vi "DS1104PlusDemo.vi"() -> ()   [LabVIEW 2018]
uses:
  <vilib>/event_ctls.llb/usereventprio.ctl
panel:
  in  "GetCurrentStatus":bool
  in  "Exit":bool
  out "错误输出":errorcluster
  in  "接口类型":u16(ring)=1 items=[""=0, "GPIB"=1, "VXI"=2, "GPIB-VXI"=3, "Serial"=4, "PXI"=5, "TCPIP"=6, "USB"=7, "FireWire"=9]
  in  "SINGLE Trigger":bool
  in  "RUN/STOP":bool
  in  "AUTO Set":bool
  in  "CLEAR Display":bool
  in  "Vertical Coupling":u16(ring) items=["AC", "DC", "Ground"]
  in  "Probe Attenuation":u16(ring) items=["1x"=1, "10x"=10]
  out "Single":bool caption="SINGLE"
  out "Normal":bool caption="NORMAL"
  out "Auto":bool caption="AUTO"
  in  "Trigger MODE":string(combo)
  in  "FORCE Trigger":bool
  in  "Trigger MENU":bool
  in  "Trigger LEVEL":dbl step=0.01 format="%.6g"
  in  "Horizontal POSITION":ext format="%#_9g"
  in  "Horizontal MENU":bool
  in  "Horizaontal SCALE":ext(ring)=1e-09 items=["1u", "2u", "5u", "10u", "20u", "50u", "100u", "200u", "500u", "1m", "2m", "5m", "10m", "20m", "50m", "100m", "200m", "500m", "1", "2", "5", "10", "20", "50", "100", "200", "500", "1000"]
  in  "Vertical SCALE":dbl(ring) items=["500u"=0.0005, "1m"=0.001, "2m"=0.002, "5m"=0.005, "10m"=0.01, "20m"=0.02, "50m"=0.05, "100m"=0.1, "200m"=0.2, "500m"=0.5, "1"=1.0, "2"=2.0, "5"=5.0, "10"=10.0, "20"=20.0, "50"=50.0, "100"=100.0]
  in  "Vertical POSITION":dbl min=-100.0 max=100.0 step=0.1 format="%#_4g"
  in  "CH4":bool
  in  "CH3":bool
  in  "CH2":bool
  in  "CH1":bool
  out "波形图":waveform(dbl)[](graph)
  in  "VISA资源名称":refnum<visa-resource-name>
  # "VERTICAL"
  # "HORIZONTAL"
  # "TRIGGER"
  # "POSITION"
  # "POSITION"
  # "V"
  # "s"
  # "SCALE"
  # "SCALE"
  # "s/div"
  # "V/div"
  # "V"
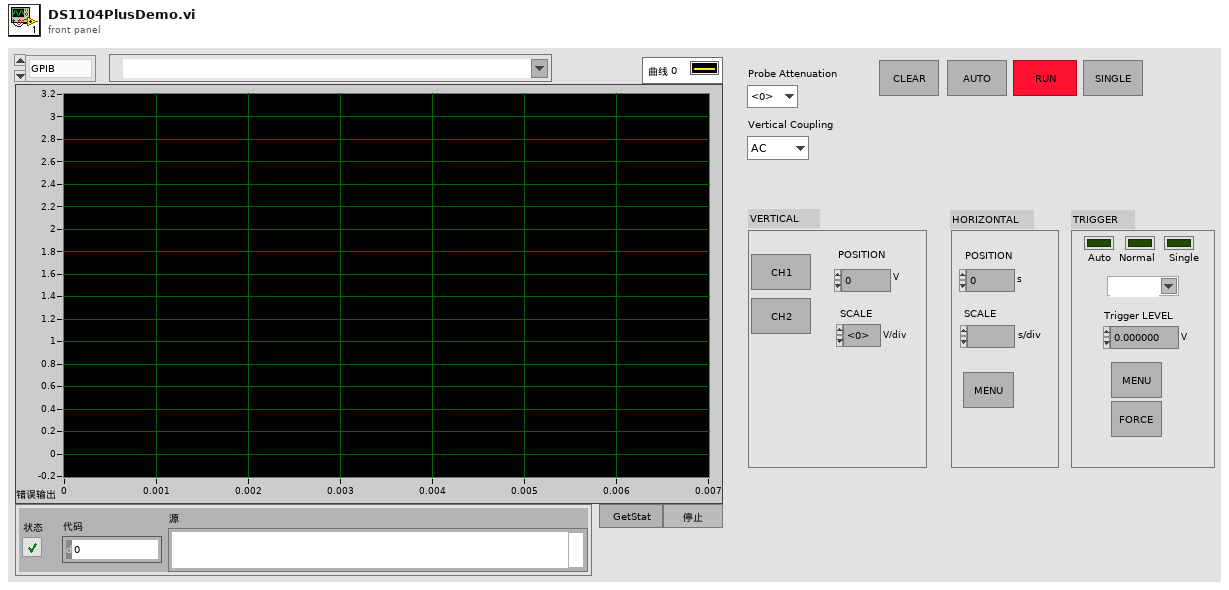
[diagram p1: front panel]
types:
  T1 = typedef "usereventprio.ctl" = enum32{"high priority", "normal priority"}
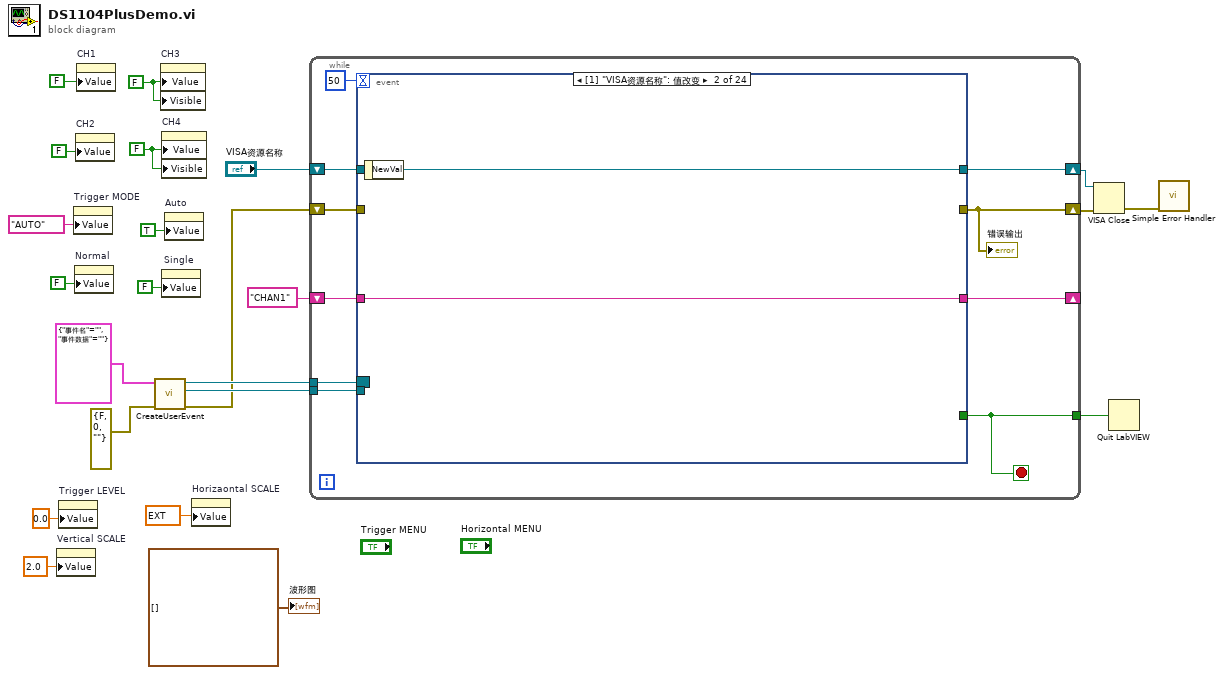
[diagram p0: block diagram]
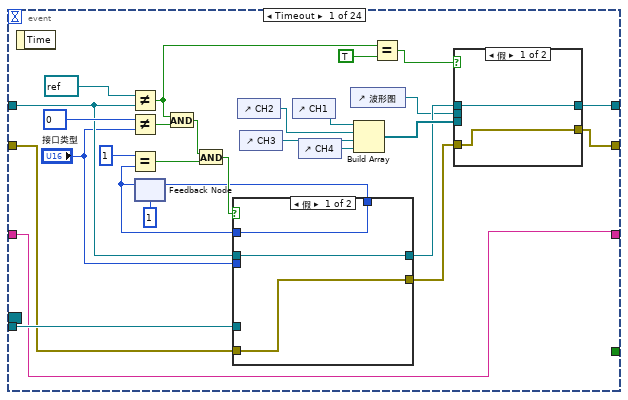
[diagram p2: hidden frame]
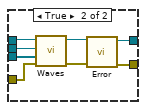
[diagram p3: hidden frame]
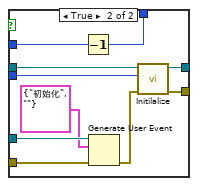
[diagram p4: hidden frame]
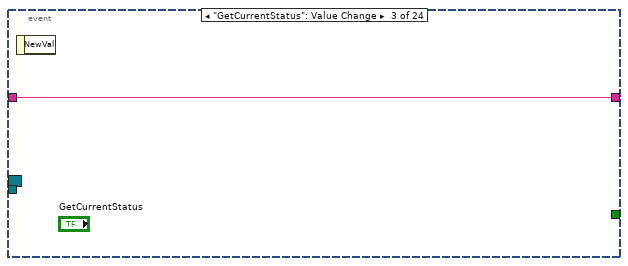
[diagram p5: hidden frame]
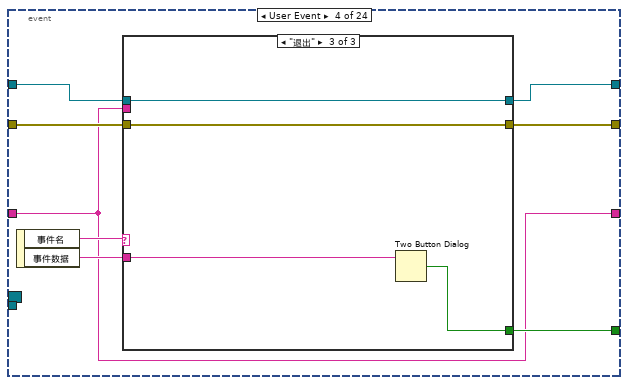
[diagram p6: hidden frame]
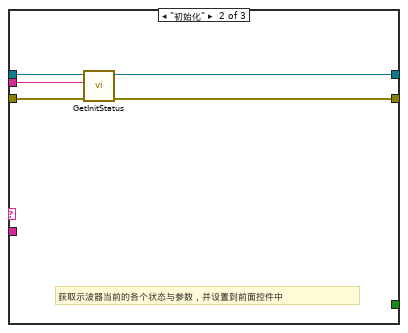
[diagram p8: hidden frame]
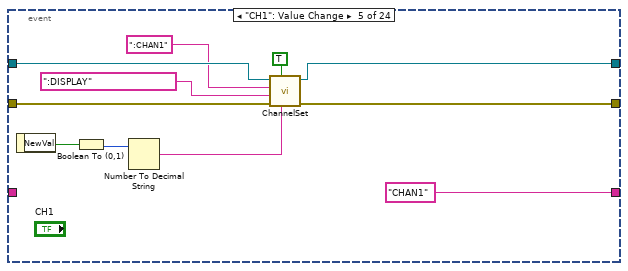
[diagram p9: hidden frame]
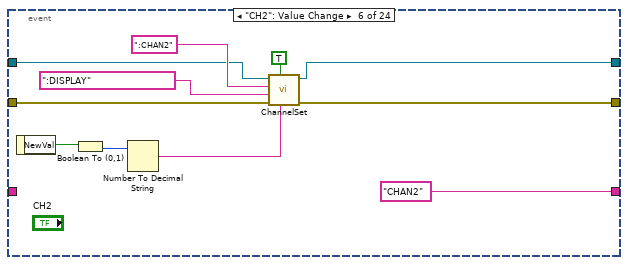
[diagram p10: hidden frame]
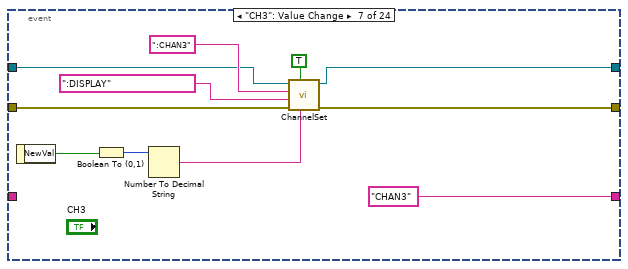
[diagram p11: hidden frame]
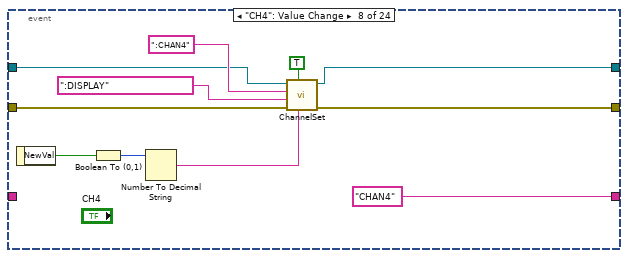
[diagram p12: hidden frame]
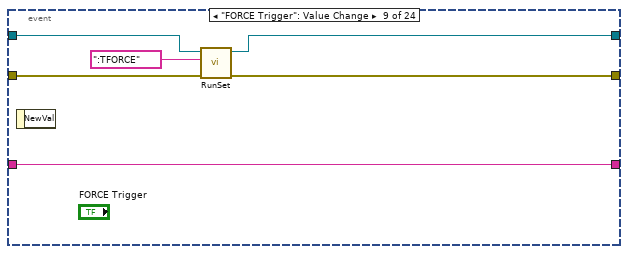
[diagram p13: hidden frame]
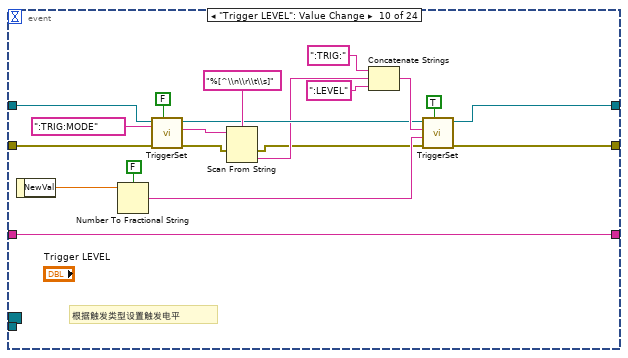
[diagram p14: hidden frame]
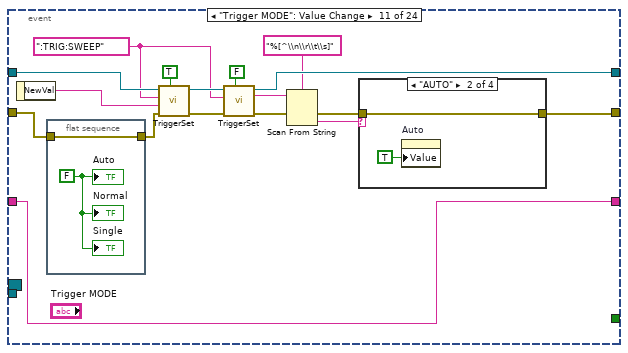
[diagram p15: hidden frame]
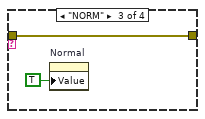
[diagram p17: hidden frame]
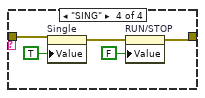
[diagram p18: hidden frame]
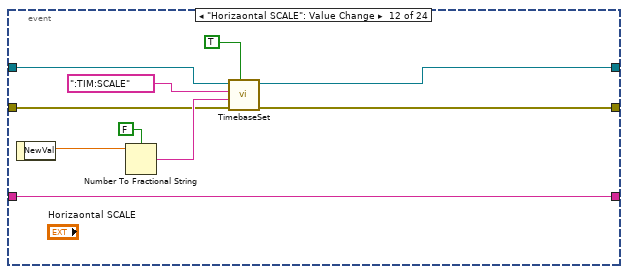
[diagram p19: hidden frame]
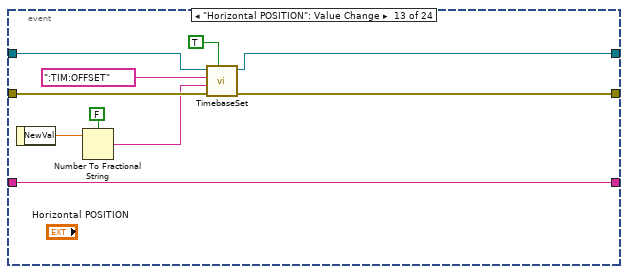
[diagram p20: hidden frame]
diagram:
  w5 = ext 0.00099999999999999999996 items=["1u", "2u", "5u", "10u", "20u", "50u", "100u", "200u", "500u", "1m", "2m", "5m", "10m", "20m", "50m", "100m", "200m", "500m", "1", "2", "5", "10", "20", "50", "100", "200", "500", "1000"] ("Horizaontal SCALE")
  w7 = 2.0 items=["500u"=0.0005, "1m"=0.001, "2m"=0.002, "5m"=0.005, "10m"=0.01, "20m"=0.02, "50m"=0.05, "100m"=0.1, "200m"=0.2, "500m"=0.5, "1"=1.0, "2"=2.0, "5"=5.0, "10"=10.0, "20"=20.0, "50"=50.0, "100"=100.0] ("Vertical SCALE")
  w8 = FALSE ("CH4")
  w9 = FALSE ("CH3")
  n1 = property on="Vertical SCALE" class="Ring (严格)"("Value"=w7) -> ()  [unwired: 2 in, 2 out]
  n2 = property on="Trigger LEVEL" class="DigNum (严格)"("Value"=0.0 ("Trigger LEVEL")) -> ()  [unwired: 2 in, 2 out]
  n3 = property on="Trigger MODE" class="CmbBox"("Value"="AUTO" ("Trigger MODE")) -> ()  [unwired: 2 in, 2 out]
  n4 = property on="Normal" class="Bool (严格)"("Value"=FALSE ("Normal")) -> ()  [unwired: 2 in, 2 out]
  n5 = property on="CH2" class="Bool (严格)"("Value"=FALSE ("CH2")) -> ()  [unwired: 2 in, 2 out]
  n6 = property on="CH1" class="Bool (严格)"("Value"=FALSE ("CH1")) -> ()  [unwired: 2 in, 2 out]
  n7 = call "CreateUserEvent.vi"("error in (no error)"=errorcluster {"status"=FALSE, "code"=0, "source"=""} ("错误常量"), "事件消息"=cluster{"事件名":string, "事件数据":string} {"事件名"="", "事件数据"=""}) -> ("error out"=w11:errorcluster, "用户事件引用句柄"=w13:refnum<user-event>, "用户事件注册引用句柄"=w14:refnum<event-registration>)  [unwired: 7 in]
  n8 = property on="CH3" class="Bool (严格)"("Value"=w9, "Visible"=w9) -> ()  [unwired: 2 in, 2 out]
  n9 = property on="CH4" class="Bool (严格)"("Value"=w8, "Visible"=w8) -> ()  [unwired: 2 in, 2 out]
  n10 = property on="Single" class="Bool (严格)"("Value"=FALSE ("Single")) -> ()  [unwired: 2 in, 2 out]
  n11 = property on="Auto" class="Bool (严格)"("Value"=TRUE ("Auto")) -> ()  [unwired: 2 in, 2 out]
  n12 = property on="Horizaontal SCALE" class="Ring (严格)"("Value"=w5) -> ()  [unwired: 2 in, 2 out]
  n13 = while {
    shift-right: [w27] -> w18
    shift-left: "VISA资源名称" -> [w32]
    shift-right: [w26] -> w17
    shift-left: w11 -> [w31]
    shift-right: [w29] -> _
    shift-left: "CHAN1" ("通道选择") -> [w30]
    tunnel: w14 -> [w25]
    tunnel: w13 -> [w28]
    tunnel: [w24] -> w1
    stop <- w24 stop-if-true
    n14 = event shown="[1] \"VISA资源名称\": 值改变" {
      selector: w25 -> [_ _ _ _ _ _ _ _ _ _ _ _ _ _ _ _ _ _ _ _ _ _ _ _]
      dyn-events: _ -> [_ _ _ _ _ _ _ _ _ _ _ _ _ _ _ _ _ _ _ _ _ _ _ _]
      timeout: 50 -> [_ _ _ _ _ _ _ _ _ _ _ _ _ _ _ _ _ _ _ _ _ _ _ _]
      tunnel: w32 -> [w46 _ _ w94 w117 w122 w135 w146 w154 w175 w193 w215 w224 w235 w243 w255 w261 w268 w274 w286 w320 w341 w358 w369]
      tunnel: w31 -> [w59 _ _ w90 w116 w121 w134 w145 w155 w174 w184 w209 w225 w226 w242 w253 w264 w267 w275 w285 w321 w340 w360 w368]
      tunnel: [w40 w85 _ w93 w109 w120 w133 w144 w151 w163 w185 w208 w219 w230 w238 w252 w262 w266 w273 w277 w315 w338 w358 w369] -> w27
      tunnel: [w37 _ _ w91 w108 w119 w132 w143 w153 w164 w186 w207 w218 w228 w237 w251 w263 w265 w272 w278 w317 w339 w359 w368] -> w26
      tunnel: w30 -> [w41 w86 w87 w88 _ _ _ _ w156 w176 w192 w206 w217 w231 w236 w249 w260 w270 w276 w287 w322 w343 w364 w370]
      tunnel: [w41 w86 w87 w88 "CHAN1" ("通道选择") "CHAN2" ("通道选择") "CHAN3" ("通道选择") "CHAN4" ("通道选择") w156 w176 w192 w206 w217 w231 w236 w249 w260 w270 w276 w287 w322 w342 w364 w370] -> w29
      tunnel: w28 -> [w60 _ _ _ _ _ _ _ _ _ _ _ _ _ _ _ _ _ _ _ _ w337 w361 _]
      tunnel: [_ _ _ w89 _ _ _ _ _ _ _ _ _ _ _ _ _ _ _ _ _ _ _ w365] -> w24
      event Timeout {
        w61 = u16 0 items=[""=0, "GPIB"=1, "VXI"=2, "GPIB-VXI"=3, "Serial"=4, "PXI"=5, "TCPIP"=6, "USB"=7, "FireWire"=9] ("接口类型")
        n15 = event-data() -> ()  [unwired: 1 in, 1 out]
        n16 = Not Equal?(x=refnum<visa-resource-name> refnum ("y"), y=w46) -> (x != y?=w35:bool)
        n17 = Not Equal?(x=w61, y="接口类型") -> (x != y?=w54:bool)
        n18 = feedback #1(1) -> (w56:i32)
        n19 = Equal?(x=1, y=w56) -> (x = y?=w53:bool)
        n20 = And(x=w35, y=w54) -> (x .and. y?=w44:bool)
        n21 = And(x=w44, y=w53) -> (x .and. y?=w52:bool)
        n22 = case shown="假" w52 {
          tunnel: w60 -> [_ w84]
          tunnel: w59 -> [w72 w82]
          tunnel: w56 -> [w74 w81]
          tunnel: [w74 w80] -> w47
          tunnel: w46 -> [w73 w79]
          tunnel: "接口类型" -> [_ w78]
          tunnel: [w73 w76] -> w42
          tunnel: [w72 w75] -> w38
          frame False {
          }
          frame True {
            n23 = Decrement(x=w81) -> (x-1=w80:i32)
            n24 = Generate User Event(user event=w84, event data cluster=cluster{"事件名":string, "事件数据":string} {"事件名"="初始化", "事件数据"=""} ("事件数据"), error in=w82) -> (error out=w77:errorcluster)  [unwired: 1 in, 1 out]
            n25 = call "Initilalize.vi"("错误输入（无错误）"=w77, "接口类型"=w78, "VISA资源名称"=w79) -> ("错误输出"=w75:errorcluster, "VISA资源名称输出"=w76:refnum<visa-resource-name>)  [unwired: 6 in, 1 out]
          }
        }
        n26 = feedback-in #1(w47) -> ()
        n27 = control-ref of="CH2"() -> (w49:refnum<vi>)
        n28 = control-ref of="CH3"() -> (w50:refnum<vi>)
        n29 = control-ref of="CH1"() -> (w48:refnum<vi>)
        n30 = control-ref of="CH4"() -> (w51:refnum<vi>)
        n31 = control-ref of="波形图"() -> (w39:refnum<vi>)
        n32 = Build Array(w48, w49, w50, w51) -> (w43:refnum<vi>[])
        n33 = Equal?(x=w35, y=TRUE) -> (x = y?=w36:bool)
        n34 = case shown="假" w36 {
          tunnel: w39 -> [_ w64]
          tunnel: w43 -> [_ w65]
          tunnel: w42 -> [w63 w67]
          tunnel: [w63 w71] -> w40
          tunnel: w38 -> [w62 w68]
          tunnel: [w62 w70] -> w37
          frame False {
          }
          frame True {
            n35 = call "Waves.vi"("error in (no error) 2"=w68, "通道使能引用数组"=w65, "波形图"=w64, "VISA资源名称输入"=w67) -> ("error out 2"=w69:errorcluster, "VISA资源名称输出"=w66:refnum<visa-resource-name>)  [unwired: 6 in]
            n36 = call "Error.vi"("error in (no error)"=w69, "VISA资源名称"=w66) -> ("错误输出"=w70:errorcluster, "VISA引用句柄输出"=w71:refnum<visa-resource-name>)  [unwired: 6 in, 2 out]
          }
        }
      }
      event "VISA资源名称": Value Change {
        n37 = event-data() -> ("NewVal"=w85:refnum<visa-resource-name>)  [unwired: 1 in]
      }
      event "GetCurrentStatus": Value Change {
        n38 = event-data() -> ()  [unwired: 1 in, 1 out]
      }
      event User Event {
        n39 = event-data() -> ("事件名"=w95:string, "事件数据"=w92:string)  [unwired: 1 in]
        n40 = case shown="\"退出\"" w95 {
          tunnel: [w96 w100 w103] -> w93
          tunnel: w94 -> [w96 w102 w103]
          tunnel: w92 -> [_ _ w106]
          tunnel: [w97 w99 w104] -> w91
          tunnel: w90 -> [w97 w101 w104]
          tunnel: [_ _ w105] -> w89
          tunnel: w88 -> [_ w98 _]
          frame Default {
          }
          frame "初始化" {
            # "获取示波器当前的各个状态与参数，并设置到前面控件中"
            n41 = call "GetInitStatus.vi"("error in (no error)"=w101, "通道选择"=w98, "VISA资源名称输入"=w102) -> ("error out"=w99:errorcluster, "VISA资源名称输出"=w100:refnum<visa-resource-name>)  [unwired: 6 in, 1 out]
          }
          frame "退出" {
            n42 = Two Button Dialog(message=w106) -> (T button?=w105:bool)  [unwired: 2 in]
          }
        }
      }
      event "CH1": Value Change {
        n43 = event-data() -> ("NewVal"=w112:bool)  [unwired: 1 in]
        n44 = Boolean To (0,1)(Boolean=w112) -> (0, 1=w111:i16)
        n45 = Number To Decimal String(number=w111) -> (decimal integer string=w110:string)  [unwired: 1 in]
        n46 = call "ChannelSet.vi"("设置参数"=w110, "参数查询(0)/设置(1)"=TRUE, "error in (no error)"=w116, "CHANNLE命令子系统"=":DISPLAY", "通道选择"=":CHAN1", "VISA资源名称"=w117) -> ("error out"=w108:errorcluster, "VISA资源名称 2"=w109:refnum<visa-resource-name>)  [unwired: 2 in, 2 out]
      }
      event "CH2": Value Change {
        n47 = event-data() -> ("NewVal"=w118:bool)  [unwired: 1 in]
        n48 = Boolean To (0,1)(Boolean=w118) -> (0, 1=w126:i16)
        n49 = Number To Decimal String(number=w126) -> (decimal integer string=w125:string)  [unwired: 1 in]
        n50 = call "ChannelSet.vi"("设置参数"=w125, "参数查询(0)/设置(1)"=TRUE, "error in (no error)"=w121, "CHANNLE命令子系统"=":DISPLAY", "通道选择"=":CHAN2", "VISA资源名称"=w122) -> ("error out"=w119:errorcluster, "VISA资源名称 2"=w120:refnum<visa-resource-name>)  [unwired: 2 in, 2 out]
      }
      event "CH3": Value Change {
        n51 = event-data() -> ("NewVal"=w130:bool)  [unwired: 1 in]
        n52 = Boolean To (0,1)(Boolean=w130) -> (0, 1=w129:i16)
        n53 = Number To Decimal String(number=w129) -> (decimal integer string=w137:string)  [unwired: 1 in]
        n54 = call "ChannelSet.vi"("设置参数"=w137, "参数查询(0)/设置(1)"=TRUE, "error in (no error)"=w134, "CHANNLE命令子系统"=":DISPLAY", "通道选择"=":CHAN3", "VISA资源名称"=w135) -> ("error out"=w132:errorcluster, "VISA资源名称 2"=w133:refnum<visa-resource-name>)  [unwired: 2 in, 2 out]
      }
      event "CH4": Value Change {
        n55 = event-data() -> ("NewVal"=w141:bool)  [unwired: 1 in]
        n56 = Boolean To (0,1)(Boolean=w141) -> (0, 1=w140:i16)
        n57 = Number To Decimal String(number=w140) -> (decimal integer string=w148:string)  [unwired: 1 in]
        n58 = call "ChannelSet.vi"("设置参数"=w148, "参数查询(0)/设置(1)"=TRUE, "error in (no error)"=w145, "CHANNLE命令子系统"=":DISPLAY", "通道选择"=":CHAN4", "VISA资源名称"=w146) -> ("error out"=w143:errorcluster, "VISA资源名称 2"=w144:refnum<visa-resource-name>)  [unwired: 2 in, 2 out]
      }
      event "FORCE Trigger": Value Change {
        n59 = event-data() -> ()  [unwired: 1 in, 1 out]
        n60 = call "RunSet.vi"("error in (no error)"=w155, "TIMEBASE命令子系统"=":TFORCE", "VISA资源名称"=w154) -> ("error out"=w153:errorcluster, "VISA资源名称 2"=w151:refnum<visa-resource-name>)  [unwired: 7 in]
      }
      event "Trigger LEVEL": Value Change {
        # "根据触发类型设置触发电平"
        n61 = event-data() -> ("NewVal"=w167:dbl)  [unwired: 1 in]
        n62 = Number To Fractional String(use system decimal point (T)=FALSE ("使用系统小数点(T)"), number=w167) -> (F-format string=w165:string)  [unwired: 2 in]
        n63 = call "TriggerSet.vi"("参数查询(0)/设置(1)"=FALSE, "error in (no error)"=w174, "TRIGGER命令子系统"=":TRIG:MODE", "VISA资源名称"=w175) -> ("error out"=w159:errorcluster, "查询返回"=w161:string, "VISA资源名称 2"=w160:refnum<visa-resource-name>)  [unwired: 4 in, 1 out]
        n64 = Scan From String(format string="%[^\\n\\r\\t\\s]" ("格式字符串"), input string=w161, error in=w159) -> (error out=w157:errorcluster, output 1=w158:string)  [unwired: 2 in, 2 out]
        n65 = Concatenate Strings(":TRIG:" ("字符串"), w158, ":LEVEL" ("字符串")) -> (w169:string)
        n66 = call "TriggerSet.vi"("参数查询(0)/设置(1)"=TRUE, "error in (no error)"=w157, "设置参数"=w165, "TRIGGER命令子系统"=w169, "VISA资源名称"=w160) -> ("error out"=w164:errorcluster, "VISA资源名称 2"=w163:refnum<visa-resource-name>)  [unwired: 3 in, 2 out]
      }
      event "Trigger MODE": Value Change {
        w187 = ":TRIG:SWEEP" ("TRIGGER命令子系统")
        n67 = event-data() -> ("NewVal"=w182:string)  [unwired: 1 in]
        n68 = flat-sequence {
          tunnel: w184 -> [w195]
          tunnel: [w195] -> w183
          frame #0 {
            w194 = FALSE
            "Auto" <- w194
            "Normal" <- w194
            "Single" <- w194
          }
        }
        n69 = call "TriggerSet.vi"("参数查询(0)/设置(1)"=TRUE, "error in (no error)"=w183, "设置参数"=w182, "TRIGGER命令子系统"=w187, "VISA资源名称"=w193) -> ("error out"=w188:errorcluster, "VISA资源名称 2"=w190:refnum<visa-resource-name>)  [unwired: 3 in, 2 out]
        n70 = call "TriggerSet.vi"("参数查询(0)/设置(1)"=FALSE, "error in (no error)"=w188, "TRIGGER命令子系统"=w187, "VISA资源名称"=w190) -> ("error out"=w180:errorcluster, "查询返回"=w181:string, "VISA资源名称 2"=w185:refnum<visa-resource-name>)  [unwired: 4 in, 1 out]
        n71 = Scan From String(format string="%[^\\n\\r\\t\\s]" ("格式字符串"), input string=w181, error in=w180) -> (error out=w178:errorcluster, output 1=w177:string)  [unwired: 2 in, 2 out]
        n72 = case shown="\"AUTO\"" w177 {
          tunnel: [w196 w197 w199 w202] -> w186
          tunnel: w178 -> [w196 w197 w199 w204]
          frame Default {
          }
          frame "AUTO" {
            n73 = property on="Auto" class="Bool (严格)"("Value"=TRUE ("Auto")) -> ()  [unwired: 2 in, 2 out]
          }
          frame "NORM" {
            n74 = property on="Normal" class="Bool (严格)"("Value"=TRUE ("Normal")) -> ()  [unwired: 2 in, 2 out]
          }
          frame "SING" {
            n75 = property on="Single" class="Bool (严格)"(error in=w204, "Value"=TRUE ("Single")) -> (error out=w203:errorcluster)  [unwired: 1 in, 1 out]
            n76 = property on="RUN/STOP" class="Bool (严格)"(error in=w203, "Value"=FALSE ("RUN/STOP")) -> (error out=w202:errorcluster)  [unwired: 1 in, 1 out]
          }
        }
      }
      event "Horizaontal SCALE": Value Change {
        n77 = event-data() -> ("NewVal"=w211:ext)  [unwired: 1 in]
        n78 = Number To Fractional String(use system decimal point (T)=FALSE ("使用系统小数点(T)"), number=w211) -> (F-format string=w210:string)  [unwired: 2 in]
        n79 = call "TimebaseSet.vi"("参数查询(0)/设置(1)"=TRUE, "error in (no error)"=w209, "设置参数"=w210, "TIMEBASE命令子系统"=":TIM:SCALE", "VISA资源名称"=w215) -> ("error out"=w207:errorcluster, "VISA资源名称 2"=w208:refnum<visa-resource-name>)  [unwired: 3 in, 2 out]
      }
      event "Horizontal POSITION": Value Change {
        n80 = event-data() -> ("NewVal"=w216:ext)  [unwired: 1 in]
        n81 = Number To Fractional String(use system decimal point (T)=FALSE ("使用系统小数点(T)"), number=w216) -> (F-format string=w220:string)  [unwired: 2 in]
        n82 = call "TimebaseSet.vi"("参数查询(0)/设置(1)"=TRUE, "error in (no error)"=w225, "设置参数"=w220, "TIMEBASE命令子系统"=":TIM:OFFSET", "VISA资源名称"=w224) -> ("error out"=w218:errorcluster, "VISA资源名称 2"=w219:refnum<visa-resource-name>)  [unwired: 3 in, 2 out]
      }
      event "Vertical SCALE": Value Change {
        n83 = event-data() -> ("NewVal"=w227:dbl)  [unwired: 1 in]
        n84 = Number To Fractional String(use system decimal point (T)=FALSE ("使用系统小数点(T)"), number=w227) -> (F-format string=w233:string)  [unwired: 2 in]
        n85 = call "ChannelSet.vi"("设置参数"=w233, "参数查询(0)/设置(1)"=TRUE, "error in (no error)"=w226, "CHANNLE命令子系统"=":SCALE", "通道选择"=w231, "VISA资源名称"=w235) -> ("error out"=w228:errorcluster, "VISA资源名称 2"=w230:refnum<visa-resource-name>)  [unwired: 2 in, 2 out]
      }
      event "Vertical POSITION": Value Change {
        n86 = event-data() -> ("NewVal"=w241:dbl)  [unwired: 1 in]
        n87 = Number To Fractional String(use system decimal point (T)=FALSE ("使用系统小数点(T)"), number=w241) -> (F-format string=w239:string)  [unwired: 2 in]
        n88 = call "ChannelSet.vi"("设置参数"=w239, "参数查询(0)/设置(1)"=TRUE, "error in (no error)"=w242, "CHANNLE命令子系统"=":OFFSET", "通道选择"=w236, "VISA资源名称"=w243) -> ("error out"=w237:errorcluster, "VISA资源名称 2"=w238:refnum<visa-resource-name>)  [unwired: 2 in, 2 out]
      }
      event "Vertical Coupling": Value Change {
        n89 = event-data() -> ("NewVal"=w248:u16)  [unwired: 1 in]
        n90 = Pick Line(multi-line string="AC\nDC\nGND" ("多行字符串"), line index=w248) -> (output string=w246:string)  [unwired: 1 in]
        n91 = call "ChannelSet.vi"("设置参数"=w246, "参数查询(0)/设置(1)"=TRUE, "error in (no error)"=w253, "CHANNLE命令子系统"=":COUPLING", "通道选择"=w249, "VISA资源名称"=w255) -> ("error out"=w251:errorcluster, "VISA资源名称 2"=w252:refnum<visa-resource-name>)  [unwired: 2 in, 2 out]
      }
      event "Probe Attenuation": Value Change {
        # "设置指定模拟通道的探头衰减比"
        n92 = event-data() -> ("NewVal"=w258:u16)  [unwired: 1 in]
        n93 = Number To Fractional String(use system decimal point (T)=FALSE ("使用系统小数点(T)"), number=w258) -> (F-format string=w256:string)  [unwired: 2 in]
        n94 = call "ChannelSet.vi"("设置参数"=w256, "error in (no error)"=w264, "CHANNLE命令子系统"=":PROBE", "通道选择"=w260, "VISA资源名称"=w261) -> ("error out"=w263:errorcluster, "VISA资源名称 2"=w262:refnum<visa-resource-name>)  [unwired: 3 in, 2 out]
      }
      event "CLEAR Display": Value Change {
        n95 = event-data() -> ()  [unwired: 1 in, 1 out]
        n96 = call "RunSet.vi"("error in (no error)"=w267, "TIMEBASE命令子系统"=":CLEAR", "VISA资源名称"=w268) -> ("error out"=w265:errorcluster, "VISA资源名称 2"=w266:refnum<visa-resource-name>)  [unwired: 7 in]
      }
      event "AUTO Set": Value Change {
        n97 = event-data() -> ()  [unwired: 1 in, 1 out]
        n98 = call "RunSet.vi"("error in (no error)"=w275, "TIMEBASE命令子系统"=":AUTOSCALE", "VISA资源名称"=w274) -> ("error out"=w272:errorcluster, "VISA资源名称 2"=w273:refnum<visa-resource-name>)  [unwired: 7 in]
      }
      event "RUN/STOP": Value Change {
        n99 = event-data() -> ("NewVal"=w281:bool)  [unwired: 1 in]
        n100 = Select(t=":RUN" ("TIMEBASE命令子系统"), s=w281, f=":STOP" ("TIMEBASE命令子系统")) -> (s? t:f=w284:string)
        n101 = call "RunSet.vi"("error in (no error)"=w285, "TIMEBASE命令子系统"=w284, "VISA资源名称"=w286) -> ("error out"=w279:errorcluster, "VISA资源名称 2"=w280:refnum<visa-resource-name>)  [unwired: 7 in]
        n102 = case shown="真" w281 {
          tunnel: w280 -> [w289 w301]
          tunnel: w279 -> [w288 w298]
          tunnel: [w288 w293] -> w278
          tunnel: [w289 w300] -> w277
          frame False {
          }
          frame True {
            n103 = property on="Single" class="Bool (严格)"(error in=w298, "Value"=FALSE ("Single")) -> (error out=w292:errorcluster)  [unwired: 1 in, 1 out]
            n104 = call "TriggerSet.vi"("参数查询(0)/设置(1)"=FALSE, "error in (no error)"=w292, "TRIGGER命令子系统"=":TRIG:SWEEP", "VISA资源名称"=w301) -> ("error out"=w296:errorcluster, "查询返回"=w290:string, "VISA资源名称 2"=w300:refnum<visa-resource-name>)  [unwired: 4 in, 1 out]
            n105 = Scan From String(format string="%[^\\n\\r\\t\\s]" ("格式字符串"), input string=w290, error in=w296) -> (error out=w294:errorcluster, output 1=w295:string)  [unwired: 2 in, 2 out]
            n106 = case shown="\"AUTO\"" w295 {
              tunnel: w294 -> [w303 w307 w310]
              tunnel: [w303 w306 w312] -> w293
              frame Default {
              }
              frame "AUTO" {
                n107 = property on="Auto" class="Bool (严格)"(error in=w307, "Value"=TRUE ("Auto")) -> (error out=w305:errorcluster)  [unwired: 1 in, 1 out]
                n108 = property on="Trigger MODE" class="CmbBox"(error in=w305, "Value"="AUTO" ("Trigger MODE")) -> (error out=w306:errorcluster)  [unwired: 1 in, 1 out]
              }
              frame "NORM" {
                n109 = property on="Trigger MODE" class="CmbBox"(error in=w310, "Value"="NORMAL" ("Trigger MODE")) -> (error out=w311:errorcluster)  [unwired: 1 in, 1 out]
                n110 = property on="Normal" class="Bool (严格)"(error in=w311, "Value"=TRUE ("Normal")) -> (error out=w312:errorcluster)  [unwired: 1 in, 1 out]
              }
            }
          }
        }
      }
      event "SINGLE Trigger": Value Change {
        n111 = event-data() -> ("NewVal"=w314:bool)  [unwired: 1 in]
        n112 = call "RunSet.vi"("error in (no error)"=w321, "TIMEBASE命令子系统"=":SINGLE", "VISA资源名称"=w320) -> ("error out"=w318:errorcluster, "VISA资源名称 2"=w316:refnum<visa-resource-name>)  [unwired: 7 in]
        n113 = case shown="真" w314 {
          tunnel: w318 -> [w323 w335]
          tunnel: [w323 w327] -> w317
          tunnel: [w324 w330] -> w315
          tunnel: w316 -> [w324 w330]
          frame False {
          }
          frame True {
            n114 = property on="Auto" class="Bool (严格)"(error in=w335, "Value"=FALSE ("Auto")) -> (error out=w334:errorcluster)  [unwired: 1 in, 1 out]
            n115 = property on="Normal" class="Bool (严格)"(error in=w334, "Value"=FALSE ("Normal")) -> (error out=w333:errorcluster)  [unwired: 1 in, 1 out]
            n116 = property on="Single" class="Bool (严格)"(error in=w333, "Value"=TRUE ("Single")) -> (error out=w329:errorcluster)  [unwired: 1 in, 1 out]
            n117 = property on="RUN/STOP" class="Bool (严格)"(error in=w329, "Value"=FALSE ("RUN/STOP")) -> (error out=w326:errorcluster)  [unwired: 1 in, 1 out]
            n118 = property on="Trigger MODE" class="CmbBox"(error in=w326, "Value"="SINGLE" ("Trigger MODE")) -> (error out=w327:errorcluster)  [unwired: 1 in, 1 out]
          }
        }
      }
      event Menu Selection (User) {
        n119 = event-data() -> ("ItemTag"=w344:string)  [unwired: 1 in]
        n120 = case shown="\"退出\"" w344 {
          tunnel: [w345 w350 w355] -> w342
          tunnel: w343 -> [w345 w350 w355]
          tunnel: w341 -> [w347 w349 w357]
          tunnel: w340 -> [w346 w353 w356]
          tunnel: [w346 w351 w356] -> w339
          tunnel: [w347 w349 w357] -> w338
          tunnel: w337 -> [_ w354 _]
          frame Default {
          }
          frame "退出" {
            n121 = Generate User Event(priority (normal)=usereventprio."high priority" ("优先级（标准）"), user event=w354, event data cluster=cluster{"事件名":string, "事件数据":string} {"事件名"="退出", "事件数据"="确定退出？"} ("事件数据"), error in=w353) -> (error out=w351:errorcluster)  [unwired: 1 out]
          }
          frame "关于" {
          }
        }
      }
      event "Exit": Value Change {
        n122 = event-data() -> ()  [unwired: 1 in, 1 out]
        n123 = Generate User Event(priority (normal)=usereventprio."high priority" ("优先级（标准）"), user event=w361, event data cluster=cluster{"事件名":string, "事件数据":string} {"事件名"="退出", "事件数据"="确定退出？"} ("事件数据"), error in=w360) -> (error out=w359:errorcluster)  [unwired: 1 out]
      }
      event Panel Close? {
        n124 = event-data() -> ()  [unwired: 1 in, 1 out]
        n125 = Two Button Dialog(message="确定退出？" ("事件数据")) -> (T button?=w365:bool)  [unwired: 2 in]
        n126 = Not(x=w365) -> (.not. x?=w366:bool)
        n127 = event-data("Discard?"=w366) -> ()  [unwired: 1 in, 1 out]
      }
    }
    "错误输出" <- w26
  }
  n128 = VISA Close(VISA resource name=w18, error in (no error)=w17) -> (error out=w2:errorcluster)
  n129 = Quit LabVIEW(quit? (T)=w1) -> ()
  n130 = call <vilib>:"Simple Error Handler.vi"("error in (no error)"=w2) -> ()  [unwired: 4 in, 5 out]
  "波形图" <- waveform(dbl)[] [] ("波形图")
